vi "Compare UDVs.vi"(8 "error in (no error)":errorcluster, 10 "UDV refs in":refnum<k21>[](array[refnum]), 11 "UDVs in":T1[](array[typedef]) {"VS ref" format="%.0x"}) -> (0 "error out":errorcluster, 2 "UDV refs out":refnum<k21>[](array[refnum]), 3 "UDVs out":T1[](array[typedef]) {"VS ref" format="%.0x"})   [LabVIEW 2019, in "Scan Engine Custom Device.lvlib"]
uses:
  Scan Engine Custom Device.lvlib
  Type Defs/UDV Data.ctl
  <vilib>/NI VeriStand/Custom Device API/Custom Device Item Ref.ctl
  Type Defs/UDV Data Type.ctl
  Type Defs/FXP Config.ctl
  Globals/Error Strings.vi
  <resource>/objmgr/ni.var.rc
  <vilib>/NI VeriStand/Custom Device API/Custom Device API.lvlib
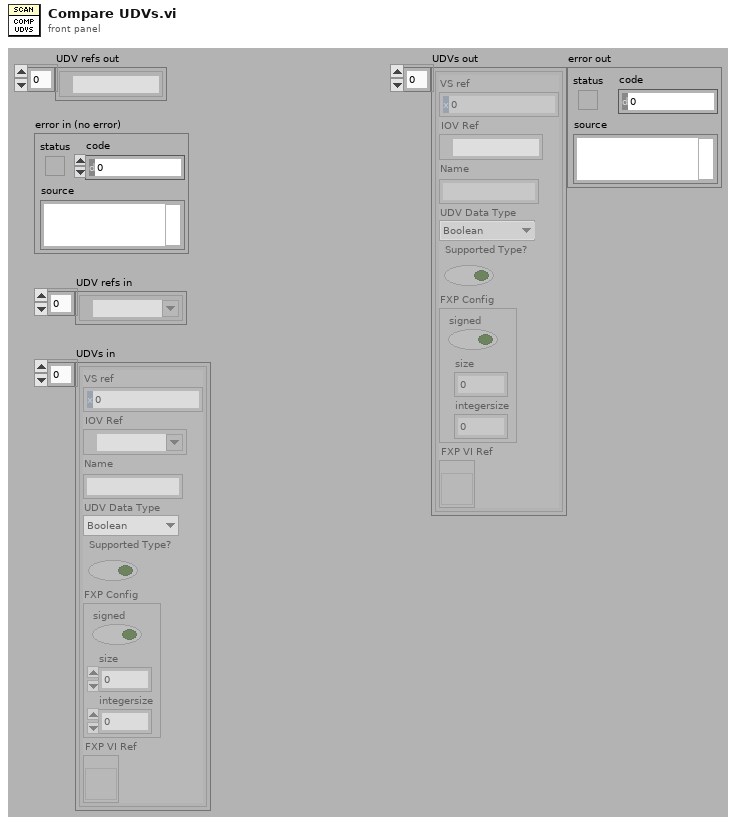
[diagram p1: front panel]
types:
  T1 = typedef "Scan Engine Custom Device.lvlib/UDV Data.ctl" = cluster{"VS ref":T2, "IOV Ref":refnum<k21>, "Name":string, "UDV Data Type":T3, "Supported Type?":bool, "FXP Config":T4, "FXP VI Ref":refnum<vi>}
  T2 = typedef "Custom Device API.lvlib/Custom Device Item Ref.ctl" = u64
  T3 = typedef "Scan Engine Custom Device.lvlib/UDV Data Type.ctl" = enum16{"Boolean", "Fixed Point", "Int8", "Int16", "Int32", "Int64", "U32 Bit Field", "UInt8", "UInt16", "UInt32", "UInt64", "Other", "DBL", "SGL"}
  T4 = typedef "Scan Engine Custom Device.lvlib/FXP Config.ctl" = cluster{"signed":bool, "size":u32, "integersize":i32}
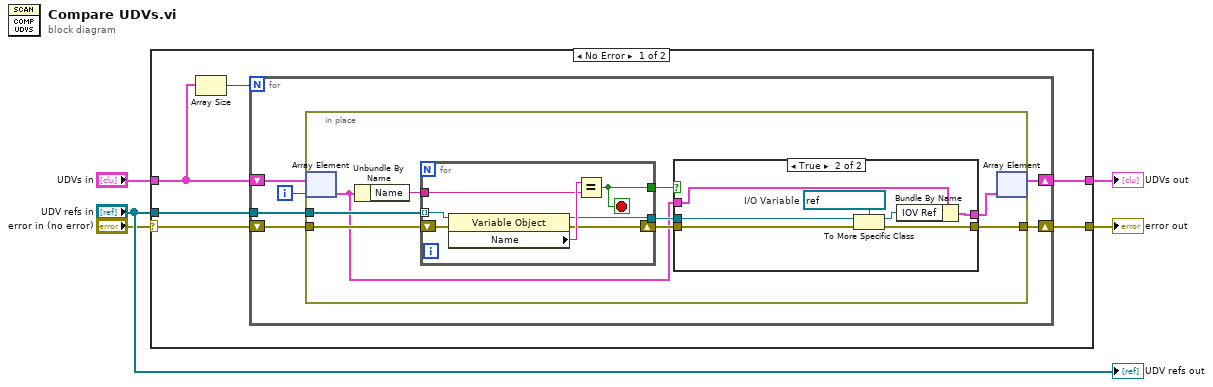
[diagram p0: block diagram]
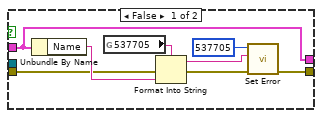
[diagram p2: hidden frame]
diagram:
  n1 = case shown="No Error" "error in (no error)" {
    selector: "error in (no error)" -> [w6 w49]
    tunnel: "UDVs in" -> [w10 w50]
    tunnel: [w9 w50] -> w4
    tunnel: [w8 w49] -> w3
    tunnel: "UDV refs in" -> [w7 _]
    frame No Error {
      n2 = Array Size(array=w10) -> (size(s)=w11:i32)
      n3 = for {
        N: w11 -> [_]
        tunnel: w7 -> [w17]
        shift-right: [w15] -> w8
        shift-left: w6 -> [w16]
        shift-right: [w12] -> w9
        shift-left: w10 -> [w13]
        i -> [w14]
        n4 = in-place {
          in-place-border: w17 -> [w26]
          in-place-border: w16 -> [w24]
          in-place-border: [w20] -> w15
          n5 = in-place-array #1(w13, w14) -> (w19:T1)
          n6 = Unbundle By Name(w19) -> ("Name"=w25:string)
          n7 = for {
            tunnel: w26 -> [w42] mode=indexing
            tunnel: w25 -> [w46]
            tunnel: [w45] -> w23
            tunnel: [w44] -> w22
            shift-right: [w43] -> w21
            shift-left: w24 -> [w48]
            stop <- w45 stop-if-true
            n8 = property class="Variable Object"(reference=w42, error in=w48) -> (reference out=w44:refnum<k21>, error out=w43:errorcluster, "Name"=w47:string)
            n9 = Equal?(x=w47, y=w46) -> (x = y?=w45:bool)
          }
          n10 = case shown="True" w23 {
            tunnel: w19 -> [w34 w41]
            tunnel: w22 -> [_ w39]
            tunnel: w21 -> [w32 w40]
            tunnel: [w29 w36] -> w20
            tunnel: [w34 w35] -> w18
            frame False {
              n11 = Unbundle By Name(w34) -> ("Name"=w33:string)
              n12 = global read "Error Strings.vi" "537705"() -> (w31:string)
              n13 = Format Into String(format string=w31, error in=w32, w33) -> (resulting string=w28:string, error out=w30:errorcluster)  [unwired: 1 in]
              n14 = call "Set Error.vi"("error in (no error)"=w30, "Message"=w28, "Code"=537705 ("error code (0)")) -> ("error out"=w29:errorcluster)  [unwired: 8 in]
            }
            frame True {
              w38 = refnum<k21> refnum  # I/O Variable
              n15 = To More Specific Class(target class=w38, reference=w39, error in=w40) -> (specific class reference=w37:refnum<k21>, error out=w36:errorcluster)
              n16 = Bundle By Name(cluster=w41, "IOV Ref"=w37) -> (w35:T1)
            }
          }
          n17 = in-place-array #1(w18) -> (w12:T1[])  [unwired: 1 out]
        }
      }
    }
    frame Error {
    }
  }
  "UDVs out" <- w4
  "error out" <- w3
  "UDV refs out" <- "UDV refs in"
